vi "FilePath.vi"() -> (0 "File Path":path)   [LabVIEW 2017, in "Configuration.lvlib"]
doc: "Returns the path to the settings file."
uses:
  Configuration.lvlib
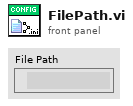
[diagram p1: front panel]
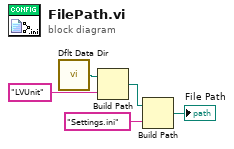
[diagram p0: block diagram]
diagram:
  n1 = call <vilib>:"Dflt Data Dir.vi"() -> ("App:Default Data Directory"=w5:path)
  n2 = Build Path(base path=w5, name or relative path="LVUnit") -> (appended path=w3:path)
  n3 = Build Path(base path=w3, name or relative path="Settings.ini") -> (appended path=→"File Path":path)
